vi "Load Node.vi"(8 "error in (no error)":errorcluster, 11 "Hot And Cold Source Unit Model in":refnum<class "Hot And Cold Source Unit Model.lvclass">) -> (0 "error out":errorcluster, 3 "Hot And Cold Source Unit Model out":refnum<class "Hot And Cold Source Unit Model.lvclass">)   [LabVIEW 2013, in "Hot And Cold Source Unit Model.lvlib" / "Hot And Cold Source Unit Model.lvclass"]
uses:
  Hot And Cold Source Unit Model.lvclass
  Hot And Cold Source Unit Model.lvclass/Hot And Cold Source Unit Model.ctl
  <vilib>/xml/Load XML File.vi
  <vilib>/xml/Close Reference(Node).vi
  <vilib>/xml/NI_XML.lvlib
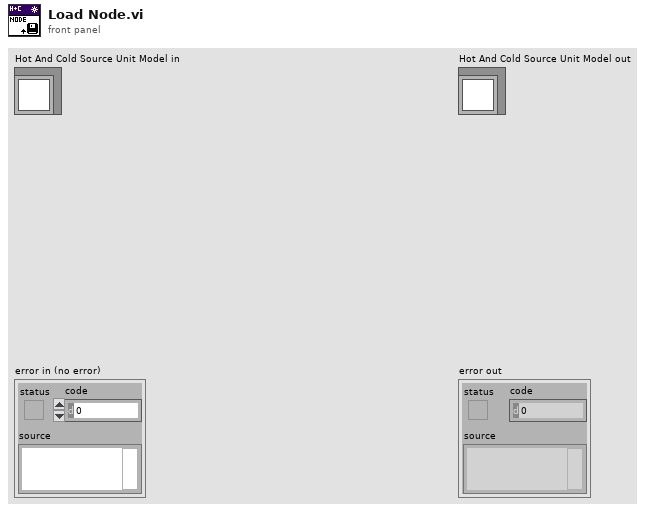
[diagram p1: front panel]
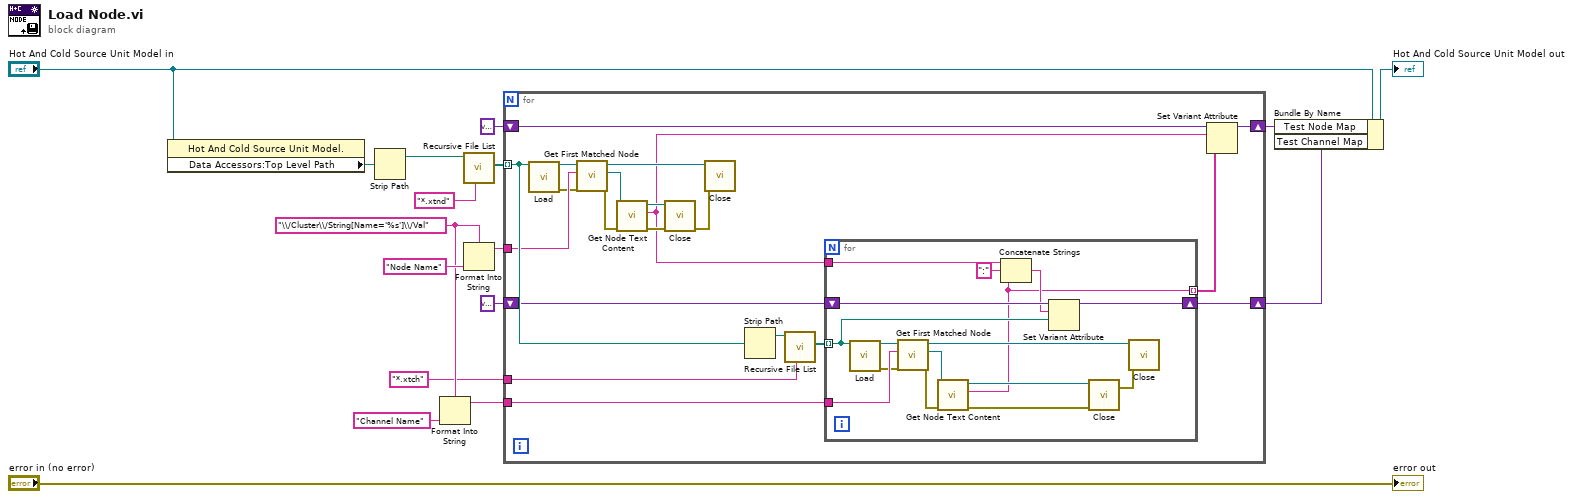
[diagram p0: block diagram]
diagram:
  w8 = "\\/Cluster\\/String[Name='%s']\\/Val" ("XPath expression")
  n1 = property class="Hot And Cold Source Unit Model."(reference="Hot And Cold Source Unit Model in") -> ("Data Accessors:Top Level Path"=w4:path)  [unwired: 1 in, 2 out]
  n2 = Strip Path(path=w4) -> (stripped path=w13:path)  [unwired: 1 out]
  n3 = Format Into String(format string=w8, "Channel Name" ("input 1")) -> (resulting string=w5:string)  [unwired: 2 in, 1 out]
  n4 = call <vilib>:"Recursive File List.vi"("pattern"="*.xtnd", "Folder Path"=w13) -> ("All Files in Dir"=w14:path[])  [unwired: 5 in, 4 out]
  n5 = Format Into String(format string=w8, "Node Name" ("input 1")) -> (resulting string=w9:string)  [unwired: 2 in, 1 out]
  n6 = for {
    tunnel: w14 -> [w30] mode=indexing
    shift-right: [w27] -> w2
    shift-left: variant -> [w26]
    shift-right: [w25] -> w3
    shift-left: variant -> [w24]
    tunnel: w9 -> [w22]
    tunnel: "*.xtch" ("pattern") -> [w20]
    tunnel: w5 -> [w19]
    n7 = call-poly <vilib>:"Load.vi"("path to XML document"=w30) -> ("DOM document out"=w34:refnum<k20>, "error out"=w21:errorcluster)  [unwired: 12 in, 1 out]
    n8 = call <vilib>:"Get First Matched Node.vi"("error in (no error)"=w21, "XPath expression"=w22, "node in"=w34) -> ("error out"=w36:errorcluster, "node result"=w37:refnum<k20>, "node out"=w32:refnum<k20>)  [unwired: 6 in]
    n9 = call <vilib>:"Get Node Text Content.vi"("error in (no error)"=w36, "node in"=w37) -> ("error out"=w33:errorcluster, "node text"=w23:string, "node out"=w35:refnum<k20>)  [unwired: 7 in]
    n10 = call-poly <vilib>:"Close.vi"("error in (no error)"=w33, "node"=w35) -> ("error out"=w31:errorcluster)  [unwired: 7 in]
    n11 = call-poly <vilib>:"Close.vi"("error in (no error)"=w31, "node"=w32) -> ()  [unwired: 7 in, 1 out]
    n12 = Strip Path(path=w30) -> (stripped path=w29:path)  [unwired: 1 out]
    n13 = call <vilib>:"Recursive File List.vi"("pattern"=w20, "Folder Path"=w29) -> ("All Files in Dir"=w28:path[])  [unwired: 5 in, 4 out]
    n14 = for {
      tunnel: w28 -> [w41] mode=indexing
      shift-right: [w46] -> w27
      shift-left: w26 -> [w45]
      tunnel: w23 -> [w44]
      tunnel: w19 -> [w40]
      tunnel: [w38] -> w18 mode=indexing
      n15 = call-poly <vilib>:"Load.vi"("path to XML document"=w41) -> ("DOM document out"=w50:refnum<k20>, "error out"=w39:errorcluster)  [unwired: 12 in, 1 out]
      n16 = call <vilib>:"Get First Matched Node.vi"("error in (no error)"=w39, "XPath expression"=w40, "node in"=w50) -> ("error out"=w48:errorcluster, "node result"=w47:refnum<k20>, "node out"=w52:refnum<k20>)  [unwired: 6 in]
      n17 = call <vilib>:"Get Node Text Content.vi"("error in (no error)"=w48, "node in"=w47) -> ("error out"=w51:errorcluster, "node text"=w38:string, "node out"=w49:refnum<k20>)  [unwired: 7 in]
      n18 = Concatenate Strings(w44, ":" ("string"), w38) -> (w43:string)
      n19 = Set Variant Attribute(Variant=w45, name=w43, value=w41) -> (Variant out=w46:variant)  [unwired: 1 in, 2 out]
      n20 = call-poly <vilib>:"Close.vi"("error in (no error)"=w51, "node"=w49) -> ("error out"=w53:errorcluster)  [unwired: 7 in]
      n21 = call-poly <vilib>:"Close.vi"("error in (no error)"=w53, "node"=w52) -> ()  [unwired: 7 in, 1 out]
    }
    n22 = Set Variant Attribute(Variant=w24, name=w23, value=w18) -> (Variant out=w25:variant)  [unwired: 1 in, 2 out]
  }
  n23 = Bundle By Name(cluster="Hot And Cold Source Unit Model in", "Test Node Map"=w3, "Test Channel Map"=w2) -> (→"Hot And Cold Source Unit Model out":refnum<class "Hot And Cold Source Unit Model.lvclass">)
  "error out" <- "error in (no error)"
